vi "Get Section 4 data.vi"(8 "error in":errorcluster, 11 "Product":string) -> (0 "error out":errorcluster, 3 "Section4":T1)   [LabVIEW 2025]
uses:
  Controls/Section4 variables.ctl
  <vilib>/Utility/config.llb/Read Key (String).vi
  <vilib>/Utility/config.llb/NI_LVConfig.lvlib
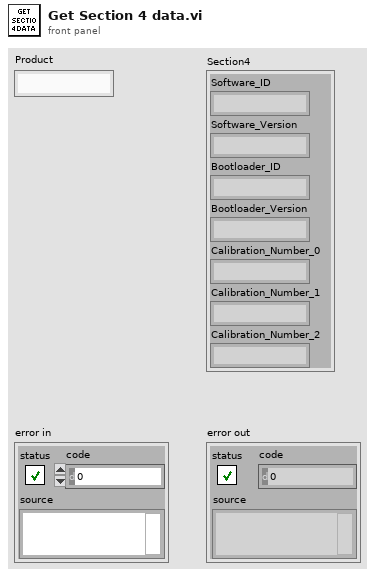
[diagram p1: front panel]
types:
  T1 = typedef "Section4 variables.ctl" = cluster{"Software_ID":string, "Software_Version":string, "Bootloader_ID":string, "Bootloader_Version":string, "Calibration_Number_0":string, "Calibration_Number_1":string, "Calibration_Number_2":string}
  T2 = typedef "NI_LVConfig.lvlib/Config Data RefNum.ctl" = refnum<k1>
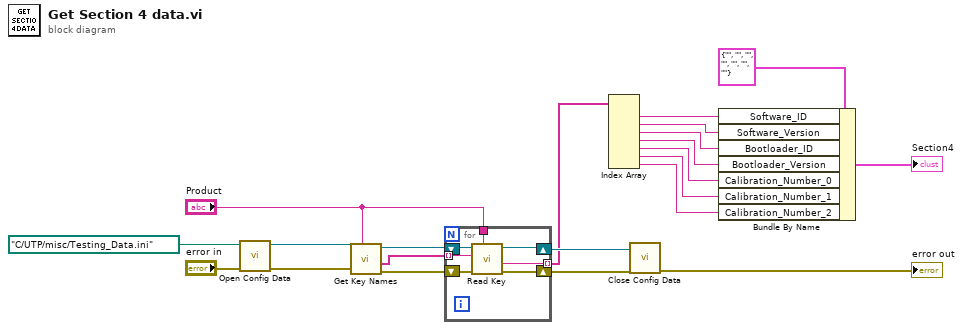
[diagram p0: block diagram]
diagram:
  n1 = call <vilib>:"Open Config Data.vi"("error in (no error)"="error in", "configuration file path"=path "C:/UTP/misc/Testing_Data.ini") -> ("error out"=w18:errorcluster, "refnum"=w19:T2)  [unwired: 7 in, 1 out]
  n2 = call <vilib>:"Get Key Names.vi"("section"="Product", "error in (no error)"=w18, "refnum"=w19) -> ("error out"=w16:errorcluster, "key names"=w14:string[], "refnum out"=w17:T2)  [unwired: 5 in, 1 out]
  n3 = for {
    tunnel: "Product" -> [w26]
    tunnel: w14 -> [w25] mode=indexing
    tunnel: [w24] -> w10 mode=indexing
    shift-right: [w23] -> w13
    shift-left: w17 -> [w28]
    shift-right: [w22] -> w12
    shift-left: w16 -> [w27]
    n4 = call-poly <vilib>:"Read Key.vi"("section"=w26, "error in (no error)"=w27, "key"=w25, "refnum"=w28) -> ("error out"=w22:errorcluster, "value"=w24:string, "refnum out"=w23:T2)  [unwired: 4 in, 1 out]
  }
  n5 = Index Array(array=w10) -> (element #1=w8:string, element #2=w7:string, element #3=w6:string, element #4=w5:string, element #5=w4:string, element #6=w3:string, element #7=w2:string)  [unwired: 7 in]
  n6 = call <vilib>:"Close Config Data.vi"("error in (no error)"=w12, "refnum"=w13) -> ("error out"=→"error out":errorcluster)  [unwired: 8 in, 1 out]
  n7 = Bundle By Name(cluster=T1 {"Software_ID"="", "Software_Version"="", "Bootloader_ID"="", "Bootloader_Version"="", "Calibration_Number_0"="", "Calibration_Number_1"="", "Calibration_Number_2"=""} ("Section4"), "Software_ID"=w8, "Software_Version"=w7, "Bootloader_ID"=w6, "Bootloader_Version"=w5, "Calibration_Number_0"=w4, "Calibration_Number_1"=w3, "Calibration_Number_2"=w2) -> (→"Section4":T1)
